vi "ultra.vi"() -> ()   [LabVIEW 2019]
uses:
  <vilib>/MakerHub/LINX/Public/Utilities/Open Serial.vi
  <vilib>/MakerHub/LINX/LMH-LINX.lvlib
panel:
  out "History Chart":dbl(graph)
  in  "Digital Input Channel":u8=13
  in  "Digital Output Channel":u8=13
  out "Centimeters":dbl(slide) scale=0.0..30.0
  in  "Serial Port":refnum<visa-resource-name>="COM3"
  in  "stop":bool
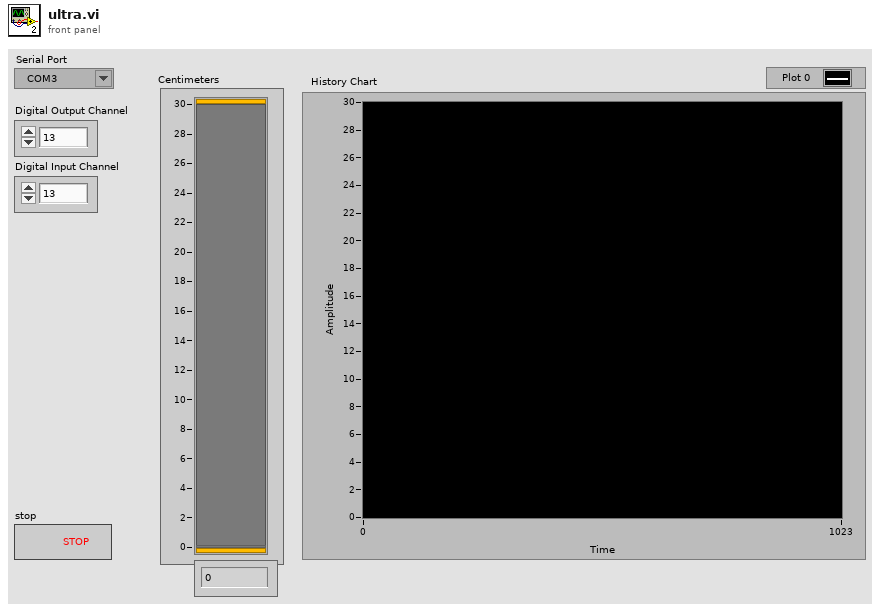
[diagram p1: front panel]
types:
  T1 = typedef "LMH-LINX.lvlib/LINX Ref.ctl" = cluster{"IO":T2, "Interface":T3, "LINX Device Config":T4}
  T2 = typedef "LMH-LINX.lvlib/Platform.ctl" = enum16{"Remote", "Local"}
  T3 = typedef "LMH-LINX.lvlib/Interface.ctl" = enum16{"Serial", "TCP"}
  T4 = typedef "LMH-LINX.lvlib/Device.lvlib/LINX Device Config.ctl" = cluster{"Interface":T3, "COM Port":refnum<visa-resource-name>, "TCP Configuration":T5, "Device Family":u8, "Device ID":u8, "Device Name":string, "TCP Ref":refnum<k5>, "Channels":T6}
  T5 = typedef "LMH-LINX.lvlib/Device.lvlib/TCP Config.ctl" = cluster{"IP Address":string, "Port":u16}
  T6 = typedef "LMH-LINX.lvlib/Channels.ctl" = cluster{"DI":u8[], "DO":u8[], "AI":u8[], "AO":u8[], "PWM":u8[], "QE":u8[], "UART":u8[], "I2C 2":u8[], "SPI":u8[], "CAN":u8[], "Servo":u8[], "AI Ref (V)":dbl, "AI Resolution (Bits)":u8, "AO Ref (V)":dbl, "AO Resolution (Bits)":u8}
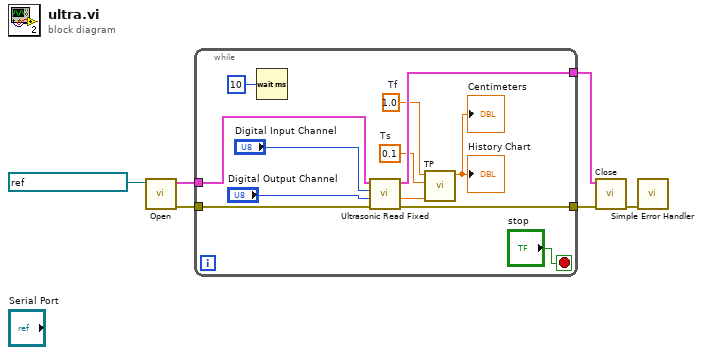
[diagram p0: block diagram]
diagram:
  n1 = call-poly <vilib>:"Open.vi"("Serial Port"=refnum<visa-resource-name> "COM3") -> ("Error Out"=w4:errorcluster, "LINX Resource"=w1:T1)  [unwired: 8 in, 1 out]
  n2 = while {
    tunnel: [w14] -> w6
    tunnel: w1 -> [w16]
    tunnel: [w13] -> w5
    tunnel: w4 -> [w15]
    stop <- "stop" stop-if-true
    w10 = 0.1  # Ts
    w9 = 1.0  # Tf
    n3 = Wait (ms)(milliseconds to wait=u32 10) -> ()  [unwired: 1 out]
    n4 = call "Ultrasonic Read Fixed.vi"("Error In"=w15, "DO Channel"="Digital Output Channel", "DI Channel"="Digital Input Channel", "LINX Resource"=w16) -> ("Error Out"=w13:errorcluster, "Centimeters"=w8:dbl, "LINX Resource"=w14:T1)  [unwired: 4 in, 1 out]
    n5 = call "TP.vi"("In_k"=w8, "Ts"=w10, "Tf"=w9) -> ("Filter out"=→"Centimeters" →"History Chart":dbl)  [unwired: 8 in]
  }
  n6 = call <vilib>:"Close.vi"("Error In"=w5, "LINX Resource"=w6) -> ("Error Out"=w3:errorcluster)  [unwired: 9 in]
  n7 = call <vilib>:"Simple Error Handler.vi"("error in (no error)"=w3) -> ()  [unwired: 4 in, 5 out]
